vi "Shut Down Device.vi"(8 "error in (no error)":errorcluster, 11 "cetoni in":refnum<class "cetoni.lvclass">) -> (0 "error out":errorcluster, 3 "cetoni out":refnum<class "cetoni.lvclass">)   [LabVIEW 2018, in "cetoni.lvlib" / "cetoni.lvclass"]
uses:
  cetoni.lvclass
  Resources/GLOBAL/GLOBAL Time-critical.vi
  Device/Device.lvclass
  <userlib>/QmixLib/QmixLib.lvlib
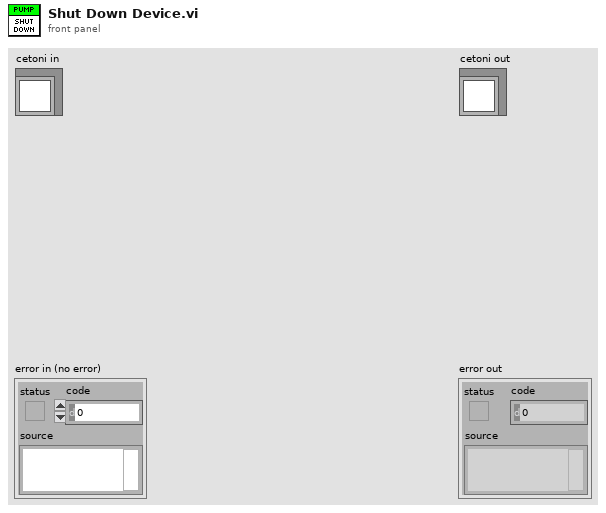
[diagram p1: front panel]
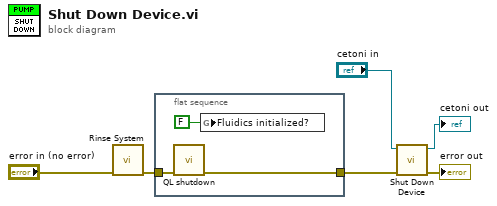
[diagram p0: block diagram]
diagram:
  n1 = call "Rinse System.vi"("error in (no error)"="error in (no error)") -> ("error out"=w1:errorcluster)  [unwired: 10 in]
  n2 = flat-sequence {
    tunnel: [w9] -> w4
    tunnel: w1 -> [w8]
    frame #0 {
      n3 = call <userlib>:"QL shutdown.vi"("error in (no error)"=w8) -> ("error out"=w9:errorcluster)  [unwired: 10 in]
      n4 = global write "GLOBAL Time-critical.vi" "Fluidics initialized?"(FALSE ("Fluidics initialized?")) -> ()
    }
  }
  n5 = call-parent "Shut Down Device.vi"("error in (no error)"=w4, "Device in"="cetoni in") -> ("error out"=→"error out":errorcluster, "Device out"=→"cetoni out":refnum<class "cetoni.lvclass">)  [unwired: 8 in]
